vi "LevyLab Instrument.Client.vi"(8 "error in (no error)":errorcluster, 9 "Data":variant, 10 "Command":T1, 11 "ExampleInstrument in":refnum<class "LevyLab Instrument.lvclass">) -> (0 "error out":errorcluster, 1 "Data out":variant, 2 "Command":string, 3 "ExampleInstrument out":refnum<class "LevyLab Instrument.lvclass">)   [LabVIEW 2016, in "LevyLab Instrument.lvclass"]
uses:
  LevyLab Instrument.lvclass
  C:/user/patrick/hg/levylab_inst/lvsrc/SMOs/Instrument/Instrument.lvclass
  Typedefs/LevyLab Instrument.Commands--Enum.ctl
  SMOs/Instrument/Instrument.lvclass
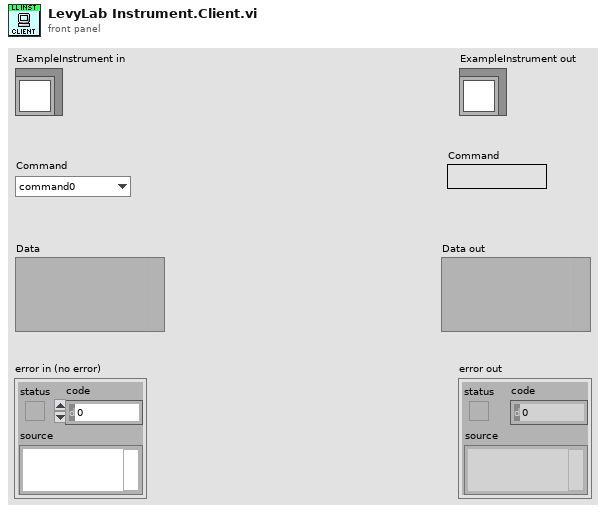
[diagram p1: front panel]
types:
  T1 = typedef "LevyLab Instrument.lvclass/LevyLab Instrument.Commands--Enum.ctl" = enum16{"command0", "command1", "command2"}
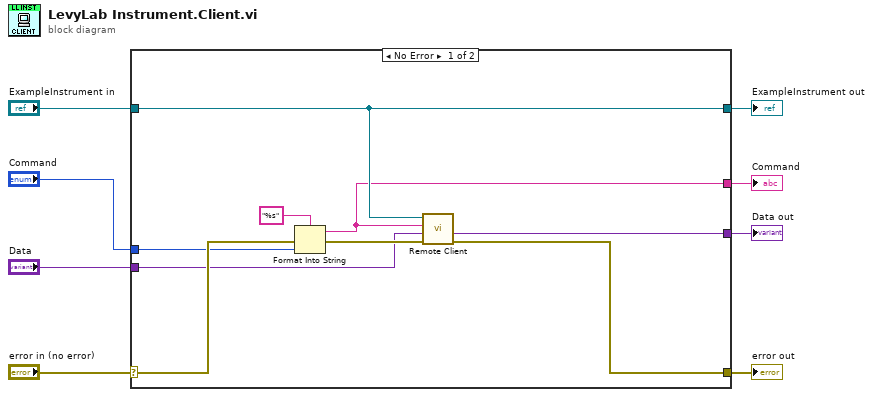
[diagram p0: block diagram]
diagram:
  n1 = case shown="No Error" "error in (no error)" {
    selector: "error in (no error)" -> [w14 w19]
    tunnel: [w13 w19] -> w7
    tunnel: [w17 w18] -> w5
    tunnel: "ExampleInstrument in" -> [w17 w18]
    tunnel: "Data" -> [w9 _]
    tunnel: "Command" -> [w12 _]
    tunnel: [w11 _] -> w2
    tunnel: [w10 _] -> w1
    frame No Error {
      n2 = Format Into String(format string="%s", error in=w14, w12) -> (resulting string=w10:string, error out=w15:errorcluster)  [unwired: 1 in]
      n3 = call "Remote Client.vi"("error in (no error)"=w15, "Data"=w9, "Command"=w10, "Instrument in"=w17) -> ("error out"=w13:errorcluster, "Data out"=w11:variant)  [unwired: 4 in, 2 out]
    }
    frame Error {
    }
  }
  "error out" <- w7
  "ExampleInstrument out" <- w5
  "Data out" <- w2
  "Command" <- w1
